vi "server.Send Shutdown Command.vi"(8 "error in (no error)":errorcluster) -> (0 "error out":errorcluster)   [LabVIEW 2016, in "JSONRPC Server.lvclass"]
doc: "This sends the following JSONRPC request:\n\n{\"jsonrpc\": \"2.0\", \"method\": \"shutdown_rpc_server\"}\n\nThe RPC Server Template contains a case that shuts down the RPC Server process when this command is received."
uses:
  JSONRPC Server.lvclass
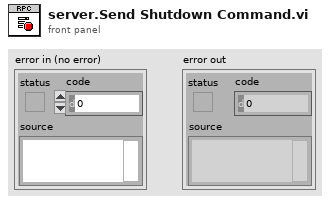
[diagram p1: front panel]
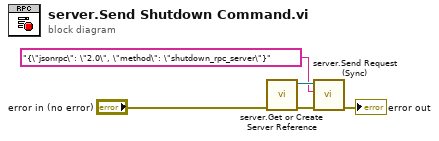
[diagram p0: block diagram]
diagram:
  n1 = call "server.Get or Create Server Reference.vi"("error in (no error)"="error in (no error)") -> ("error out"=w2:errorcluster, "Server Out"=w5:refnum<class "JSONRPC Server.lvclass">)  [unwired: 9 in]
  n2 = call "server.Send Request (Sync).vi"("error in (no error)"=w2, "JSON Request String"="{\"jsonrpc\": \"2.0\", \"method\": \"shutdown_rpc_server\"}", "JSONRPC Server in"=w5) -> ("error out"=→"error out":errorcluster)  [unwired: 6 in, 2 out]
